vi "d2.6 (hw1).vi"() -> ()   [LabVIEW 2017]
panel:
  out "Surface Area":dbl
  out "Volume":dbl
  in  "Sphere Diameter":dbl
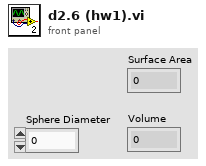
[diagram p1: front panel]
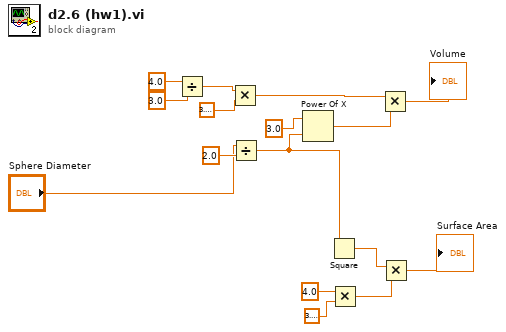
[diagram p0: block diagram]
diagram:
  n1 = Divide(x=4.0, y=3.0) -> (x/y=w14:dbl)
  n2 = Multiply(x=w14, y=3.141592653589793) -> (x*y=w10:dbl)
  n3 = Divide(x="Sphere Diameter", y=2.0) -> (x/y=w4:dbl)
  n4 = Power Of X(1:w4, 2:3.0 ("y")) -> (0:w9:dbl)
  n5 = Square(x=w4) -> (x^2=w3:dbl)
  n6 = Multiply(x=4.0, y=3.141592653589793) -> (x*y=w2:dbl)
  n7 = Multiply(x=w10, y=w9) -> (x*y=→"Volume":dbl)
  n8 = Multiply(x=w3, y=w2) -> (x*y=→"Surface Area":dbl)
